vi "fg_data_re-shared.vi"(1 "initialize?":bool) -> (0 "data out":dbl)   [LabVIEW 2015, in "lv_mutex_shared_1.lvlib"]
uses:
  lv_mutex_shared_1.lvlib
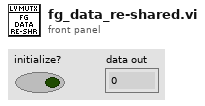
[diagram p1: front panel]
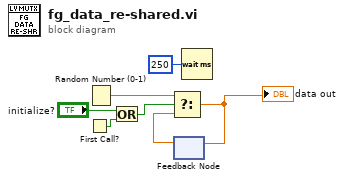
[diagram p0: block diagram]
diagram:
  n1 = First Call?() -> (First Call?: T/F=w2:bool)
  n2 = Random Number (0-1)() -> (number: 0 to 1=w1:dbl)
  n3 = Or(x="initialize?", y=w2) -> (x .or. y?=w4:bool)
  n4 = feedback #1() -> (w6:dbl)  [unwired: 1 in]
  n5 = Select(t=w1, s=w4, f=w6) -> (s? t:f=w7:dbl)
  "data out" <- w7
  n6 = feedback-in #1(w7) -> ()
  n7 = Wait (ms)(milliseconds to wait=u32 250) -> ()  [unwired: 1 out]
